vi "my data to share.vi"(11 "Data interval (s)":dbl) -> (3 "Shared Data":T1 {"scaled" format="%.2f"})   [LabVIEW 2015]
uses:
  shared data (name value unit).ctl
  DAQ configuration/Sensor buffer command.ctl
  Process Controller 3.0/logic buffer cmd.ctl
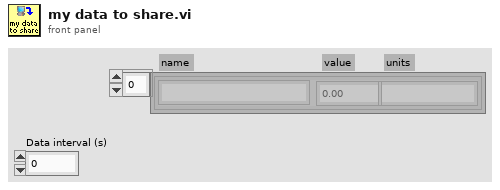
[diagram p1: front panel]
types:
  T1 = typedef "shared data (name value unit).ctl" = cluster{"name":string, "units":string, "scaled":sgl}[]
  T2 = typedef "logic buffer cmd.ctl" = enum16{"read", "write ouput settings", "write rules", "write setpoints", "write output descriptions", "write all", "calculate setpoints", "save", "open", "Load all setpoint code", "Load one setpoint code", "Configure one setpoint code"}
  T3 = typedef "Sensor buffer command.ctl" = enum16{"read average", "read recent", "read all", "write", "set buffer size", "Read channel config", "Write channel config", "clear"}
  T4 = typedef "Sensor data.ctl" = cluster{" Sensor array":T5[], "Time":dbl}
  T5 = typedef "sensor cluster.ctl" = cluster{"voltage":sgl, "scaled":sgl, "units":string, "Out of Range":bool}
  T6 = typedef "Channel config.ctl" = cluster{"Channel Indices":T7[], "AI Max voltage":dbl[], "Calibration matrix":T8}
  T7 = typedef "channel identifier.ctl" = u16
  T8 = typedef "calib array.ctl" = T9[]
  T9 = typedef "conversion.ctl" = cluster{"conversion matrix":sgl[][], "units":string, "name":string, "scale type":T10, "offset (volts)":dbl, "second channel":i8, "correspondence table":T11, "offset (physical units)":dbl, "pH scale":T12, "D.O.":T13, "Photometer data":T14}
  T10 = typedef "scale type.ctl" = enum16{"Volts", "Polynomial", "Correspondence Table", "pH", "Dissolved Oxygen", "Quadratic", "Photometer"}
  T11 = typedef "correspondence table.ctl" = cluster{"physical units":dbl, "volts":dbl}[]
  T12 = typedef "pH scale.ctl" = cluster{"Buffers":cluster{"Buffer":dbl, "Calibrated":bool, "V/T":dbl}[], "Temperature":dbl}
  T13 = typedef "DO scale.ctl" = cluster{"Temperature":dbl, "K":dbl, "barometric pressure":dbl}
  T14 = typedef "Photometer calibration data.ctl" = cluster{"Dark Voltage":dbl, "Blank Voltage":dbl, "Standards":cluster{"Concentration":dbl, "Voltage":dbl}[]}
  T15 = cluster{"name":string, "units":string, "scaled":sgl}
  T16 = typedef "variable setpoint.ctl" = cluster{"name":string, "unit":string, "value":dbl, "Type":enum16{"Constant", "Variable"}, "variable":cluster{"selected sensors":i32[], "selected set points":i32[], "VI":path, "Data average interval":T17, "code ref":T18}}
  T17 = typedef "data ave interval.ctl" = dbl
  T18 = typedef "type specifier for control code.ctl" = refnum<vi>
  T19 = cluster{"name":string, "units":string, "scaled":sgl}[]
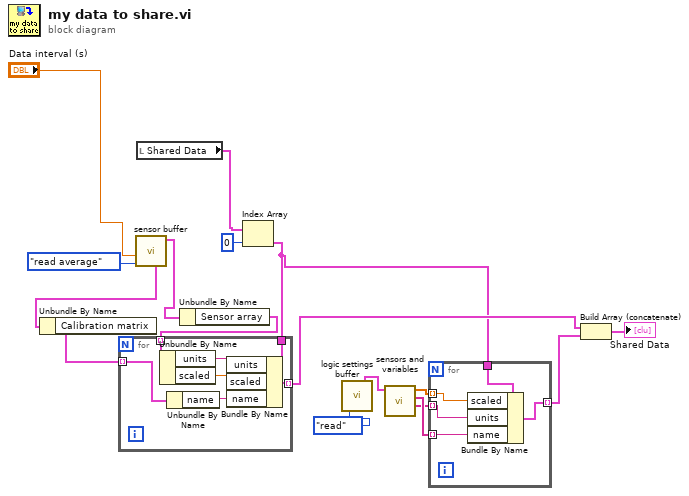
[diagram p0: block diagram]
diagram:
  n1 = call "sensor buffer.vi"("command"=Sensor_buffer_command."read average", "smooth interval (s)"="Data interval (s)") -> ("Calibrated data"=w9:T4, "Channel Config out"=w7:T6)  [unwired: 5 in, 3 out]
  n2 = Unbundle By Name(w7) -> ("Calibration matrix"=w8:T8)
  n3 = local read "Shared Data"() -> (w1:T1)
  n4 = Unbundle By Name(w9) -> ("Sensor array"=w10:T5[])
  n5 = Index Array(array=w1, index=0) -> (element=w12:T15)
  n6 = for {
    tunnel: w8 -> [w19] mode=indexing
    tunnel: w10 -> [w24] mode=indexing
    tunnel: [w21] -> w14 mode=indexing
    tunnel: w12 -> [w20]
    n7 = Unbundle By Name(w24) -> ("units"=w23:string, "scaled"=w22:sgl)
    n8 = Unbundle By Name(w19) -> ("name"=w18:string)
    n9 = Bundle By Name(cluster=w20, "units"=w23, "scaled"=w22, "name"=w18) -> (w21:T15)
  }
  n10 = call "logic settings buffer.vi"("command"=logic_buffer_cmd."read") -> ("Set Points out"=w4:T16[])  [unwired: 11 in, 7 out]
  n11 = call "sensors and variables.vi"("S P & V definitions"=w4) -> ("units"=w6:string[], "Variable names"=w13:string[], "Variable values"=w5:dbl[])  [unwired: 6 in, 2 out]
  n12 = for {
    tunnel: w12 -> [w29]
    tunnel: w5 -> [w28] mode=indexing
    tunnel: w6 -> [w27] mode=indexing
    tunnel: [w26] -> w15 mode=indexing
    tunnel: w13 -> [w25] mode=indexing
    n13 = Bundle By Name(cluster=w29, "scaled"=w28, "units"=w27, "name"=w25) -> (w26:T15)
  }
  n14 = Build Array (concatenate)(w14, w15) -> (→"Shared Data":T19)
